vi "spill_param_tcp_client.vi"(6 "n_try":i32=2, 7 "wait_time":i32=100, 8 "port":u16=9999, 9 "address":string="127.0.0.1") -> (0 "status":bool, 1 "spill_id":i32=-1, 2 "EOS":bool, 3 "BOS":bool)   [LabVIEW 2019]
panel:
  out "client_step":i32
  out "error out":errorcluster
  # "Preallocated clone reentrant execution"
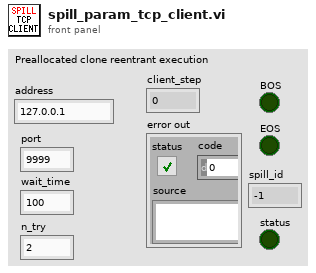
[diagram p1: front panel]
types:
  T1 = enum16{"Standard", "Buffered", "CRLF", "Immediate"}
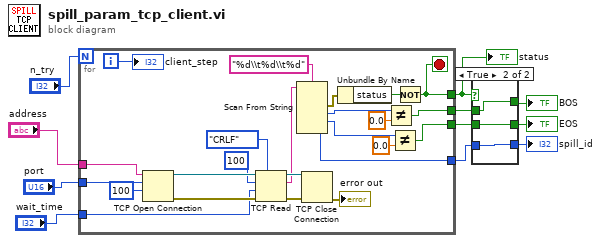
[diagram p0: block diagram]
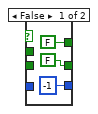
[diagram p2: hidden frame]
diagram:
  n1 = for {
    N: "n_try" -> [_]
    tunnel: [w26] -> w9
    tunnel: [w23] -> w7
    tunnel: [w20] -> w6
    tunnel: [w19] -> w5
    tunnel: "address" -> [w18]
    tunnel: "port" -> [w17]
    tunnel: "wait_time" -> [w12]
    i -> [w28]
    stop <- w26 stop-if-true
    n2 = TCP Open Connection(address=w18, remote port or service name=w17, timeout ms (60000)=100) -> (connection ID=w16:refnum<k5>, error out=w15:errorcluster)  [unwired: 2 in]
    n3 = TCP Read(connection ID=w16, bytes to read=100, error in (no error)=w15, 7:T1."CRLF" ("mode (standard)"), 9:w12) -> (connection ID out=w34:refnum<k5>, data out=w32:string, error out=w35:errorcluster)
    n4 = Scan From String(format string="%d\\t%d\\t%d", input string=w32) -> (error out=w30:errorcluster, output 1=w24:i32, output 2=w21:i32, output 3=w19:i32)  [unwired: 5 in, 2 out]
    n5 = TCP Close Connection(connection ID=w34, error in (no error)=w35) -> (error out=→"error out":errorcluster)  [unwired: 1 in, 1 out]
    n6 = Unbundle By Name(w30) -> ("status"=w27:bool)
    n7 = Not Equal?(x=w24, y=0.0) -> (x != y?=w23:bool)
    n8 = Not Equal?(x=w21, y=0.0) -> (x != y?=w20:bool)
    n9 = Not(x=w27) -> (.not. x?=w26:bool)
    "client_step" <- w28
  }
  "status" <- w9
  n10 = case shown="True" w9 {
    tunnel: [-1 w41] -> w10
    tunnel: w5 -> [_ w41]
    tunnel: [FALSE w40] -> w4
    tunnel: [FALSE w39] -> w8
    tunnel: w7 -> [_ w40]
    tunnel: w6 -> [_ w39]
    frame False {
    }
    frame True {
    }
  }
  "spill_id" <- w10
  "BOS" <- w4
  "EOS" <- w8
